vi "Check for Empty Data.vi"(11 "F0 Array (Labial)":dbl[](array[numeric])) -> (3 "spreadsheet string":string)   [LabVIEW 2020]
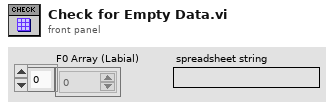
[diagram p1: front panel]
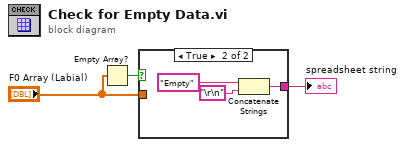
[diagram p0: block diagram]
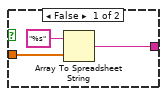
[diagram p2: hidden frame]
diagram:
  n1 = Empty Array?(array="F0 Array (Labial)") -> (empty?=w3:bool)
  n2 = case shown="True" w3 {
    tunnel: [w5 w8] -> w1
    tunnel: "F0 Array (Labial)" -> [w4 _]
    frame False {
      n3 = Array To Spreadsheet String(array=w4, 3:"%s" ("format string")) -> (spreadsheet string=w5:string)  [unwired: 1 in]
    }
    frame True {
      n4 = Concatenate Strings("Empty" ("spreadsheet string"), "\r\n") -> (w8:string)
    }
  }
  "spreadsheet string" <- w1
